vi "FF_compute2333.vi"(6 "CenVel":dbl[](array[numeric]), 7 "DesiredM_FF":dbl[](array[numeric])=[5.0, 5.0, 5.0, 4.0, 4.0, 4.0], 10 "CenPt":dbl[](array[numeric]), 11 "Array":T1[](array[typedef])) -> (0 "Closest Pt":dbl[](array[numeric]), 3 "ForceXYZ":dbl[](array[numeric]), 4 "curr Point":dbl[](array[numeric]), 5 "DesiredFM_FF":dbl[](array[numeric]))   [LabVIEW 2013]
uses:
  typeDef/AnkleTraj.ctl
  <vilib>/Analysis/_algsub.llb/Real Vector Norm.vi
  <vilib>/Analysis/baseanly.llb/Real Dot Product.vi
  <vilib>/Analysis/BLAS.llb/idamin - Min Element Index (DBL).vi
  <vilib>/Analysis/NI_AALBase.lvlib
  <vilib>/Analysis/NI_AALPro.lvlib
  <vilib>/Analysis/NI_AALBLAS.lvlib
panel:
  out "HalfWindow FF":i32
  out "P'":dbl[](array[numeric])
  out "Array 4":dbl[](array[numeric])
  out "OrderOfClosePt":i32
  out "P1":dbl[][](array[numeric])
  in  "Array 2":dbl[](array[numeric])=[0.0, 0.05, 0.0]
  in  "Enum":enum16{"Linear", "Bell"}(ring)=enum."Bell"
  out "ForceComp":dbl[](array[numeric])
  out "n_dir":dbl[](array[numeric])
  out "d_min":dbl
  out "TangentVectorAtClosestPt":dbl[](array[numeric])
  out "NormalVectorToClosestPt":dbl[](array[numeric])
  out "DistanceToClosestPt":dbl
  out "IndexOfClosePt":i32
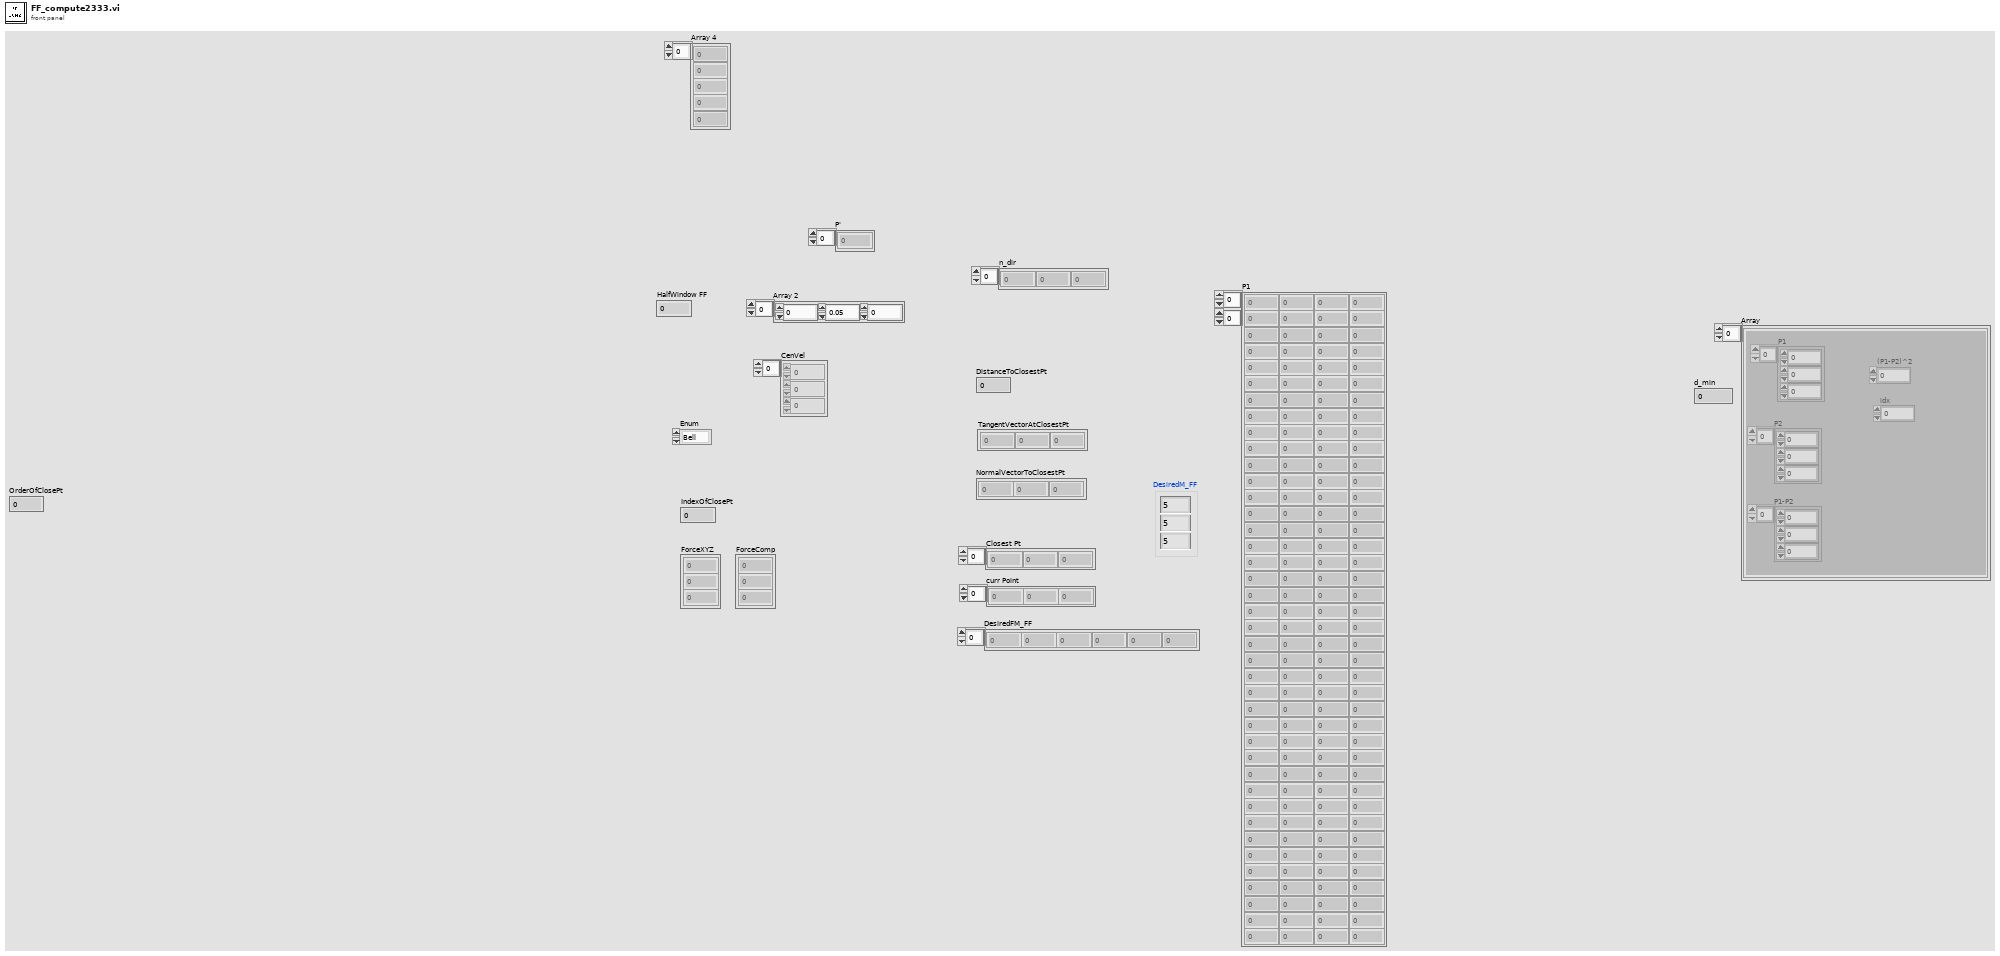
[diagram p1: front panel]
types:
  T1 = typedef "AnkleTraj.ctl" = cluster{"P1":dbl[], "P2":dbl[], "P1-P2":dbl[], "(P1-P2)^2":dbl, "idx":i32}
  T2 = cluster{"Kn":dbl, "Kt":dbl, "Kd":dbl, "Dn":dbl, "Dt":dbl}
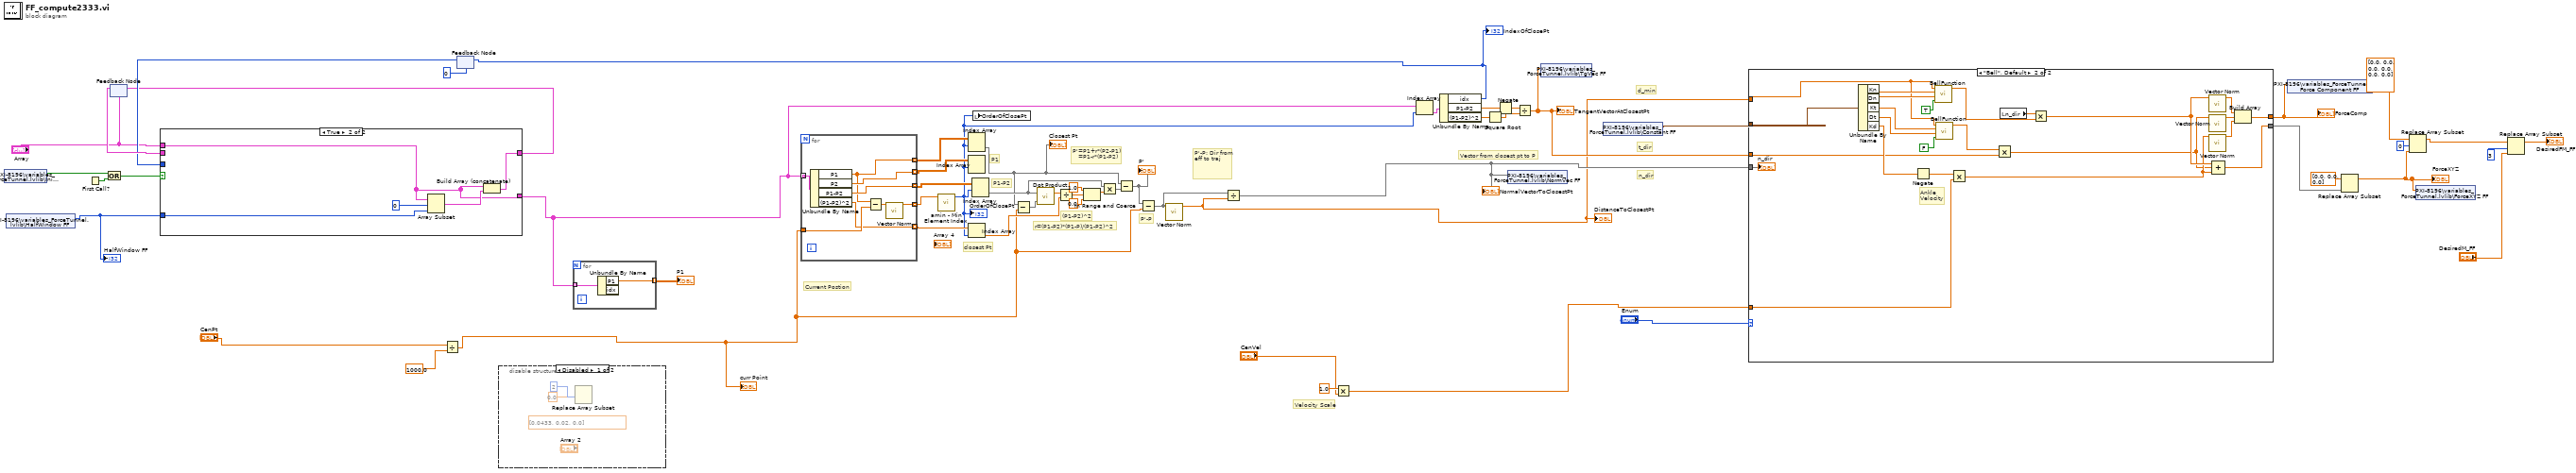
[diagram p0: block diagram]
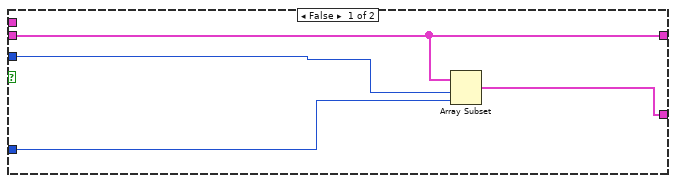
[diagram p2: hidden frame]
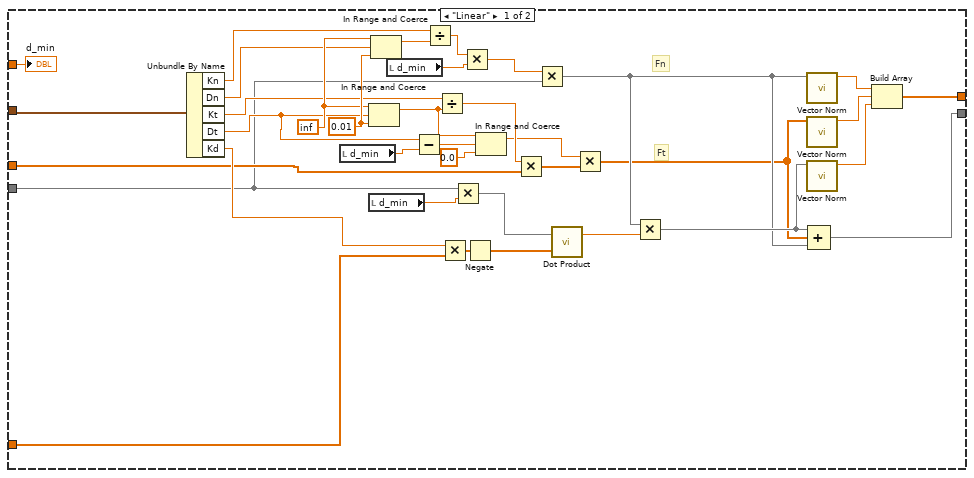
[diagram p4: hidden frame]
diagram:
  # "(P1-P2)^2"
  # "closest Pt"
  # "P1-P2"
  # "P1"
  # "P'-P"
  # "P'-P: Dir from eff to traj"
  # "r=(P1-P2)*(P1-P)/(P1-P2)^2"
  # "P'=P1+r*(P2-P1)\n   =P1-r*(P1-P2)"
  # "Current Postion"
  # "Velocity Scale"
  # "t_dir"
  # "n_dir"
  # "d_min"
  # "Vector from closest pt to P"
  n1 = shared-variable "PXI-8196\\variables_ForceTunnel.lvlib\\Init FF"() -> (w1:bool)  [unwired: 1 in, 1 out]
  n2 = shared-variable "PXI-8196\\variables_ForceTunnel.lvlib\\HalfWindow FF"() -> (w24:i32)  [unwired: 1 in, 1 out]
  "HalfWindow FF" <- w24
  n3 = First Call?() -> (First Call?: T/F=w55:bool)
  n4 = Or(x=w1, y=w55) -> (x .or. y?=w54:bool)
  n5 = feedback #1("Array") -> (w53:T1[])
  n6 = Divide(x="CenPt", y=1000.0) -> (x/y=w2:dbl[])
  "curr Point" <- w2
  n7 = feedback #2(0) -> (w52:i32)
  n8 = case shown="True" w54 {
    tunnel: w52 -> [w57 _]
    tunnel: w53 -> [w60 _]
    tunnel: [w59 w63] -> w30
    tunnel: [w60 w64] -> w32
    tunnel: "Array" -> [_ w63]
    tunnel: w24 -> [w58 w62]
    frame False {
      n9 = Array Subset(array=w60, index=w57, length=w58) -> (w59:T1[])
    }
    frame True {
      n10 = Array Subset(array=w63, index=0, length=w62) -> (w65:T1[])
      n11 = Build Array (concatenate)(w63, w65) -> (w64:T1[])
    }
  }
  n12 = feedback-in #1(w32) -> ()
  n13 = disable-structure shown="Disabled" {
    frame Disabled {
      (unwired) dbl[] [0.0433, 0.02, 0.0]
      n14 = Replace Array Subset(new element=0.0 ("new element/subarray"), index=2) -> ()  [unwired: 1 in, 1 out]
    }
    frame Enabled {
    }
  }
  n15 = for {
    tunnel: w30 -> [w69] mode=indexing
    tunnel: [w68] -> w31 mode=indexing
    n16 = Unbundle By Name(w69) -> ("P1"=w68:dbl[])  [unwired: 1 out]
  }
  "P1" <- w31
  n17 = for {
    tunnel: w30 -> [w77] mode=indexing
    tunnel: w2 -> [w74]
    tunnel: [w73] -> w12 mode=indexing
    tunnel: [w76] -> w11 mode=indexing
    tunnel: [w75] -> w10 mode=indexing
    tunnel: [w72] -> w9 mode=indexing
    tunnel: [w70] -> w3 mode=indexing
    n18 = Unbundle By Name(w77) -> ("P1"=w73:dbl[], "P2"=w76:dbl[], "P1-P2"=w75:dbl[], "(P1-P2)^2"=w72:dbl)
    n19 = Subtract(x=w73, y=w74) -> (x-y=w71:dbl[])
    n20 = call-poly <vilib>:"Vector Norm.vi"("Input Vector"=w71) -> ("norm"=w70:dbl)  [unwired: 9 in, 1 out]
  }
  n21 = call-poly <vilib>:"amin - Min Element Index.vi"("x"=w3) -> ("idamin"=w7:i32)  [unwired: 9 in, 1 out]
  "OrderOfClosePt" <- w7
  n22 = Index Array(array=w12, index (row)=w7) -> (element=w8:dbl[])  [unwired: 1 in]
  "Closest Pt" <- w8
  n23 = Index Array(array=w9, index=w7) -> (element=w16:dbl)
  n24 = Index Array(array=w11, index (row)=w7) -> ()  [unwired: 1 in, 1 out]
  n25 = Index Array(array=w10, index (row)=w7) -> (element=w15:dbl[])  [unwired: 1 in]
  n26 = local write "OrderOfClosePt"(w7) -> ()
  n27 = Subtract(x=w8, y=w2) -> (x-y=w23:dbl[])
  n28 = call-poly <vilib>:"Dot Product.vi"("Y Vector"=w23, "X Vector"=w15) -> ("X * Y"=w22:dbl)  [unwired: 1 out]
  n29 = Divide(x=w22, y=w16) -> (x/y=w21:dbl)
  n30 = In Range and Coerce(upper limit=1.0, x=w21, lower limit=0.0) -> (coerced(x)=w18:dbl)  [unwired: 1 out]
  n31 = Multiply(x=w15, y=w18) -> (x*y=w17:dbl[])
  n32 = Subtract(x=w8, y=w17) -> (x-y=w13:dbl[])
  "P'" <- w13
  n33 = Subtract(x=w13, y=w2) -> (x-y=w14:dbl[])
  n34 = call-poly <vilib>:"Vector Norm.vi"("Input Vector"=w14) -> ("norm"=w4:dbl)  [unwired: 9 in, 1 out]
  "DistanceToClosestPt" <- w4
  n35 = Divide(x=w14, y=w4) -> (x/y=w6:dbl[])
  "NormalVectorToClosestPt" <- w6
  n36 = Multiply(x=1.0, y="CenVel") -> (x*y=w48:dbl[])
  n37 = Index Array(array=w30, index=w7) -> (element=w42:T1)
  n38 = Unbundle By Name(w42) -> ("idx"=w5:i32, "P1-P2"=w45:dbl[], "(P1-P2)^2"=w46:dbl)
  "IndexOfClosePt" <- w5
  n39 = feedback-in #2(w5) -> ()
  n40 = Square Root(x=w46) -> (sqrt(x)=w44:dbl)
  n41 = Negate(x=w45) -> (-x=w43:dbl[])
  n42 = shared-variable "PXI-8196\\variables_ForceTunnel.lvlib\\NormVec FF"(w6) -> ()  [unwired: 1 in, 1 out]
  n43 = Divide(x=w43, y=w44) -> (x/y=w25:dbl[])
  "TangentVectorAtClosestPt" <- w25
  n44 = shared-variable "PXI-8196\\variables_ForceTunnel.lvlib\\TgVec FF"(w25) -> ()  [unwired: 1 in, 1 out]
  n45 = shared-variable "PXI-8196\\variables_ForceTunnel.lvlib\\Constant FF"() -> (w26:T2)  [unwired: 1 in, 1 out]
  n46 = case shown="\"Bell\", Default" "Enum" {
    tunnel: [w113 w130] -> w27
    tunnel: [w92 w137] -> w47
    tunnel: w48 -> [w112 w134]
    tunnel: w26 -> [w91 w128]
    tunnel: w25 -> [w85 w119]
    tunnel: w4 -> [w83 w116]
    tunnel: w6 -> [w84 w118]
    frame "Linear" {
      w97 = inf
      w98 = 0.01 ("upper limit")
      # "Ft"
      # "Fn"
      n47 = Unbundle By Name(w91) -> ("Kn"=w90:dbl, "Dn"=w89:dbl, "Kt"=w88:dbl, "Dt"=w87:dbl, "Kd"=w86:dbl)
      n48 = local read "d_min"() -> (w81:dbl)
      n49 = In Range and Coerce(upper limit=w97, x=w87, lower limit=w98) -> (coerced(x)=w99:dbl)  [unwired: 1 out]
      n50 = local read "d_min"() -> (w80:dbl)
      n51 = In Range and Coerce(upper limit=w97, x=w89, lower limit=w98) -> (coerced(x)=w100:dbl)  [unwired: 1 out]
      n52 = local read "d_min"() -> (w82:dbl)
      n53 = Subtract(x=w87, y=w81) -> (x-y=w103:dbl)
      n54 = Divide(x=w90, y=w100) -> (x/y=w96:dbl)
      n55 = Divide(x=w88, y=w99) -> (x/y=w101:dbl)
      n56 = Multiply ("Multiply.vi")(x=w86, y=w112) -> (x*y=w108:dbl[])
      n57 = Multiply(x=w84, y=w80) -> (x*y=w107:dbl[])
      n58 = Multiply(x=w96, y=w82) -> (x*y=w95:dbl)
      n59 = Negate(x=w108) -> (-x=w106:dbl[])
      n60 = In Range and Coerce(upper limit=w99, x=w103, lower limit=0.0) -> (coerced(x)=w78:dbl)  [unwired: 1 out]
      n61 = Multiply(x=w101, y=w85) -> (x*y=w104:dbl[])
      n62 = Multiply(x=w95, y=w84) -> (x*y=w93:dbl[])
      n63 = call-poly <vilib>:"Dot Product.vi"("Y Vector"=w106, "X Vector"=w107) -> ("X * Y"=w105:dbl)  [unwired: 1 out]
      n64 = Multiply(x=w78, y=w104) -> (x*y=w79:dbl[])
      n65 = Multiply(x=w93, y=w105) -> (x*y=w94:dbl[])
      n66 = call-poly <vilib>:"Vector Norm.vi"("Input Vector"=w93) -> ("norm"=w109:dbl)  [unwired: 9 in, 1 out]
      n67 = call-poly <vilib>:"Vector Norm.vi"("Input Vector"=w79) -> ("norm"=w110:dbl)  [unwired: 9 in, 1 out]
      n68 = call-poly <vilib>:"Vector Norm.vi"("Input Vector"=w94) -> ("norm"=w111:dbl)  [unwired: 9 in, 1 out]
      n69 = Compound Arithmetic op=ADD(w94, w79, w93) -> (w92:dbl[])
      n70 = Build Array(w109, w110, w111) -> (w113:dbl[])
      "d_min" <- w83
    }
    frame "Bell", Default {
      # "Ankle\nVelocity"
      n71 = Unbundle By Name(w128) -> ("Kn"=w121:dbl, "Dn"=w122:dbl, "Kt"=w123:dbl, "Dt"=w124:dbl, "Kd"=w127:dbl)
      n72 = Negate(x=w127) -> (-x=w129:dbl)
      n73 = call "BellFunction.vi"("Invert"=TRUE, "(r)adius"=w122, "(A)mplitude"=w121, "x"=w116) -> ("y"=w114:dbl)  [unwired: 2 in]
      n74 = call "BellFunction.vi"("Invert"=FALSE, "(r)adius"=w124, "(A)mplitude"=w123, "x"=w116) -> ("y"=w120:dbl)  [unwired: 2 in]
      n75 = Multiply(x=w129, y=w134) -> (x*y=w135:dbl[])
      n76 = Multiply(x=w120, y=w119) -> (x*y=w115:dbl[])
      n77 = local read "n_dir"() -> (w117:dbl[])
      n78 = Multiply(x=w117, y=w114) -> (x*y=w136:dbl[])
      n79 = call-poly <vilib>:"Vector Norm.vi"("Input Vector"=w136) -> ("norm"=w133:dbl)  [unwired: 9 in, 1 out]
      n80 = call-poly <vilib>:"Vector Norm.vi"("Input Vector"=w115) -> ("norm"=w132:dbl)  [unwired: 9 in, 1 out]
      n81 = call-poly <vilib>:"Vector Norm.vi"("Input Vector"=w135) -> ("norm"=w131:dbl)  [unwired: 9 in, 1 out]
      n82 = Compound Arithmetic op=ADD(w136, w115, w135) -> (w137:dbl[])
      n83 = Build Array(w133, w132, w131) -> (w130:dbl[])
      "n_dir" <- w118
    }
  }
  "ForceComp" <- w27
  n84 = shared-variable "PXI-8196\\variables_ForceTunnel.lvlib\\Force Component FF"(w27) -> ()  [unwired: 1 in, 1 out]
  n85 = Replace Array Subset(array=dbl[] [0.0, 0.0, 0.0], new element=w47) -> (w28:dbl[])  [unwired: 1 in]
  "ForceXYZ" <- w28
  n86 = Replace Array Subset(array=dbl[] [0.0, 0.0, 0.0, 0.0, 0.0, 0.0] ("element"), new element=w28, index=0) -> (w35:dbl[])
  n87 = shared-variable "PXI-8196\\variables_ForceTunnel.lvlib\\ForceXYZ FF"(w28) -> ()  [unwired: 1 in, 1 out]
  n88 = Replace Array Subset(array=w35, new element="DesiredM_FF", index=3) -> (→"DesiredFM_FF":dbl[])
